vi "test_struct_ads_volume.vi"() -> ()   [LabVIEW 2017]
doc: "Minimal example that demonstrates functions implemented in the SorpPropLib for adsorption working pairs based on the volumetric approach and using the vapor pressure as additional property."
panel:
  out "Der. of loading wrt. pressure":cluster{dbl[], dbl[]}[](graph)
  out "Der. of loading wrt. temperature":cluster{dbl[], dbl[]}[](graph)
  out "Der. of pressure wrt. loading":cluster{dbl[], dbl[]}[](graph)
  out "Der. of pressure wrt. temperature":cluster{dbl[], dbl[]}[](graph)
  out "Temperature":cluster{dbl[], dbl[]}[](graph)
  out "Pressure":cluster{dbl[], dbl[]}[](graph)
  out "Loading":cluster{dbl[], dbl[]}[](graph)
  in  "WorkingPair (Input)":T1={"no_iso"=1, "no_p_sat"=1, "path_db"="D:\\Driesel\\SorpLibLocal\\labview_wrapper\\data\\json\\sorpproplib.json", "wp_as"="silica gel pellet", "wp_st"="123", "wp_iso"="DubininArctan1", "wp_rf"="Water", "rf_rhol"="SaturatedLiquidDensity_EoS1", "no_rhol"=1, "rf_psat"="VaporPressure_EoS1"}
  in  "Temperature in K (Input)":dbl=300.0
  in  "Pressure in Pa (Input)":dbl=1000.0
  # "Increase pressure by 5000 Pa in steps of 1 Pa."
  # "Path to database"
  # "Name of sorbent"
  # "Name of sub-type of sorbent"
  # "Name of refrigerant"
  # "Name of isotherm"
  # "ID of isotherm"
  # "Name of calculation approach for vapor pressure"
  # "ID of vapor pressure equation"
  # "Name of calculation approach for liquid density"
  # "ID of liquid density equation"
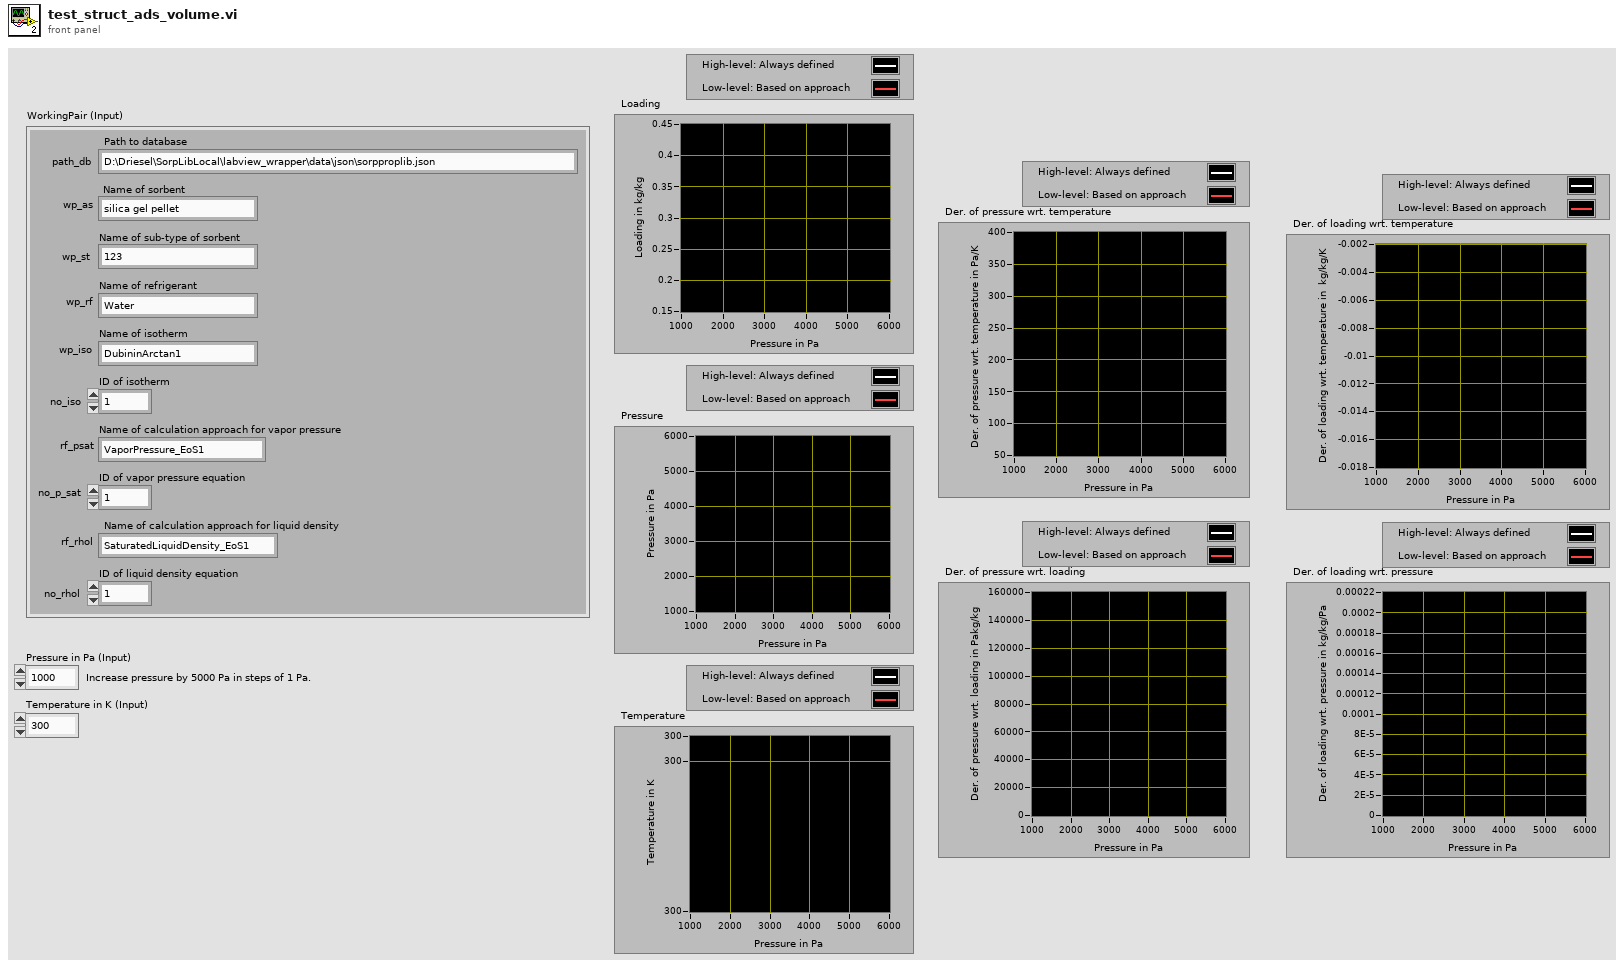
[diagram p1: front panel]
types:
  T1 = cluster{"no_iso":i32, "no_p_sat":i32, "path_db":string, "wp_as":string, "wp_st":string, "wp_iso":string, "wp_rf":string, "rf_rhol":string, "no_rhol":i32, "rf_psat":string}
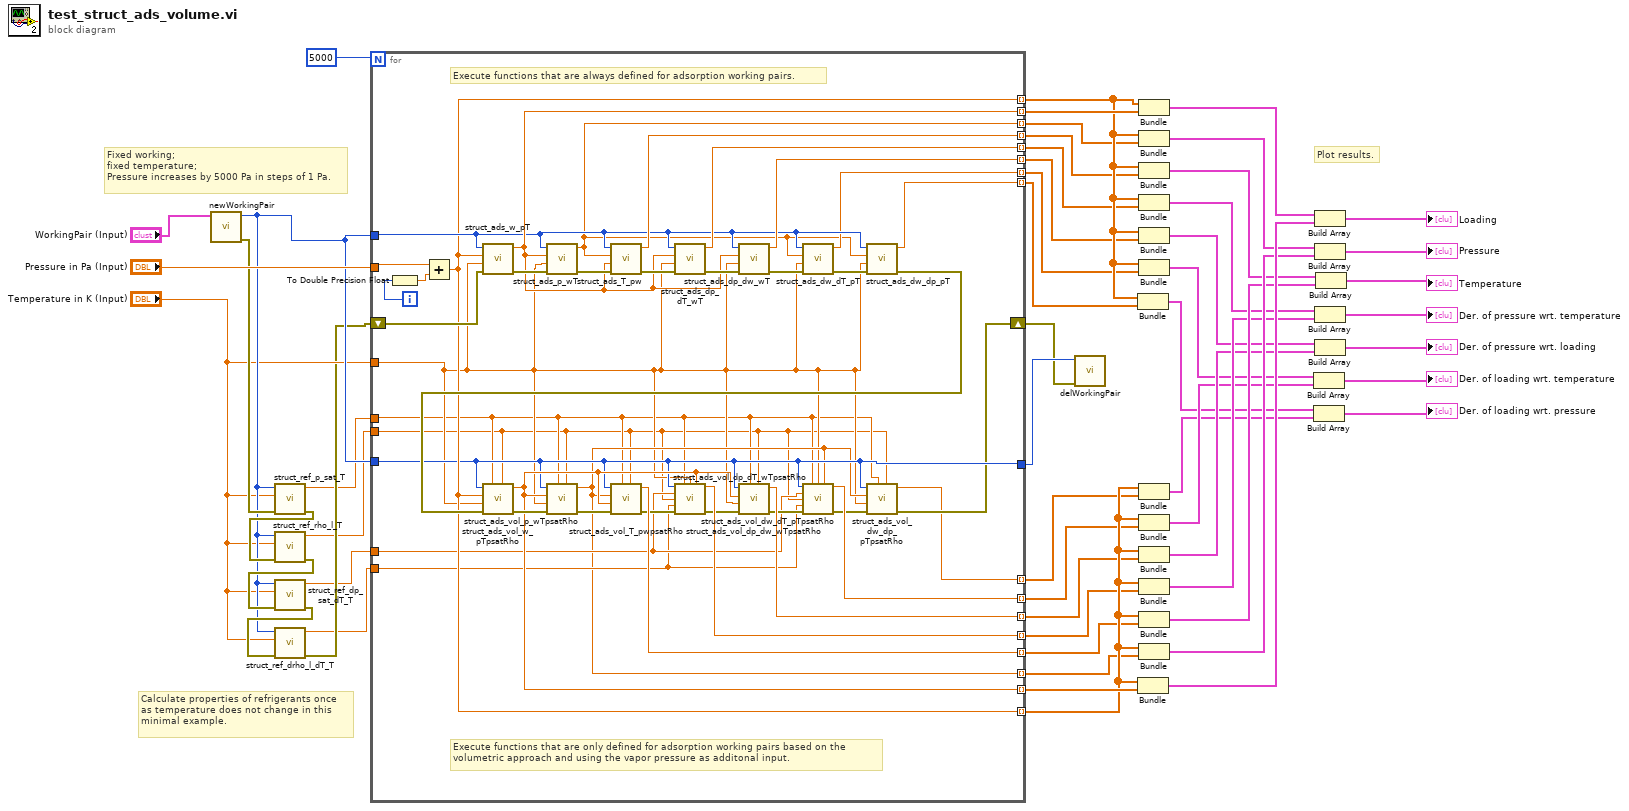
[diagram p0: block diagram]
diagram:
  # "Calculate properties of refrigerants once\nas temperature does not change in this\nminimal example."
  # "Plot results."
  # "Fixed working;\nfixed temperature;\nPressure increases by 5000 Pa in steps of 1 Pa."
  n1 = call "newWorkingPair.vi"("WorkingPair (Input)"="WorkingPair (Input)") -> ("Error (Output)"=w11:errorcluster, "workingPair"=w7:i64)  [unwired: 9 in]
  n2 = call "struct_ref_p_sat_T.vi"("Error (Input)"=w11, "Temperature in K (Input)"="Temperature in K (Input)", "Reference working pair (Input)"=w7) -> ("Error (Output)"=w10:errorcluster, "Saturation pressure in Pa (Output)"=w4:dbl)  [unwired: 7 in]
  n3 = call "struct_ref_rho_l_T.vi"("Error (Input)"=w10, "Temperature in K (Input)"="Temperature in K (Input)", "Reference working pair (Input)"=w7) -> ("Error (Output)"=w9:errorcluster, "Saturated liquid density in kg/m3 (Output)"=w3:dbl)  [unwired: 7 in]
  n4 = call "struct_ref_dp_sat_dT_T.vi"("Error (Input)"=w9, "Temperature in K (Input)"="Temperature in K (Input)", "Reference working pair (Input)"=w7) -> ("Error (Output)"=w8:errorcluster, "Der. of saturation pressure wrt temperature in Pa/K (Output)"=w2:dbl)  [unwired: 7 in]
  n5 = call "struct_ref_drho_l_dT_T.vi"("Error (Input)"=w8, "Temperature in K (Input)"="Temperature in K (Input)", "Reference working pair (Input)"=w7) -> ("Error (Output)"=w5:errorcluster, "Der. of saturated liquid density wrt temperature in kg/m3/K (Output)"=w1:dbl)  [unwired: 7 in]
  n6 = for {
    N: 5000 -> [_]
    tunnel: "Pressure in Pa (Input)" -> [w93]
    tunnel: "Temperature in K (Input)" -> [w59]
    tunnel: w7 -> [w79]
    shift-right: [w55] -> w12
    shift-left: w5 -> [w90]
    tunnel: [w88] -> w48 mode=indexing
    tunnel: [w74] -> w50 mode=indexing
    tunnel: [w81] -> w51 mode=indexing
    tunnel: [w76] -> w49 mode=indexing
    tunnel: [w86] -> w47 mode=indexing
    tunnel: [w83] -> w46 mode=indexing
    tunnel: [w78] -> w44 mode=indexing
    tunnel: [w77] -> w45 mode=indexing
    tunnel: w7 -> [w61]
    tunnel: [w67] -> w43 mode=indexing
    tunnel: [w74] -> w42 mode=indexing
    tunnel: [w60] -> w41 mode=indexing
    tunnel: [w72] -> w40 mode=indexing
    tunnel: [w70] -> w29 mode=indexing
    tunnel: [w66] -> w26 mode=indexing
    tunnel: [w62] -> w22 mode=indexing
    tunnel: [w54] -> w21 mode=indexing
    tunnel: [w61] -> w13
    tunnel: w4 -> [w58]
    tunnel: w3 -> [w57]
    tunnel: w2 -> [w64]
    tunnel: w1 -> [w63]
    i -> [w92]
    # "Execute functions that are only defined for adsorption working pairs based on the\nvolumetric approach and using the vapor pressure as additonal input."
    # "Execute functions that are always defined for adsorption working pairs."
    n7 = To Double Precision Float(number=w92) -> (double precision float=w91:dbl)
    n8 = Add(x=w93, y=w91) -> (x+y=w74:dbl)
    n9 = call "struct_ads_w_pT.vi"("Error (Input)"=w90, "Temperature in K (Input)"=w59, "Pressure in Pa (Input)"=w74, "Reference working pair (Input)"=w79) -> ("Error (Output)"=w89:errorcluster, "Loading in kg/kg (Output)"=w81:dbl)  [unwired: 6 in]
    n10 = call "struct_ads_p_wT.vi"("Error (Input)"=w89, "Temperature in K (Input)"=w59, "Loading in kg/kg (Input)"=w81, "Reference working pair (Input)"=w79) -> ("Error (Output)"=w87:errorcluster, "Pressure in Pa (Output)"=w76:dbl)  [unwired: 6 in]
    n11 = call "struct_ads_T_pw.vi"("Error (Input)"=w87, "Loading in kg/kg (Input)"=w81, "Pressure in Pa (Input)"=w76, "Reference working pair (Input)"=w79) -> ("Error (Output)"=w85:errorcluster, "Temperature in K (Output)"=w88:dbl)  [unwired: 6 in]
    n12 = call "struct_ads_dp_dT_wT.vi"("Error (Input)"=w85, "Temperature in K (Input)"=w59, "Loading in kg/kg (Input)"=w81, "Reference working pair (Input)"=w79) -> ("Error (Output)"=w84:errorcluster, "Der. of pressure wrt. temperature in Pa/K (Output)"=w86:dbl)  [unwired: 6 in]
    n13 = call "struct_ads_dp_dw_wT.vi"("Error (Input)"=w84, "Temperature in K (Input)"=w59, "Loading in kg/kg (Input)"=w81, "Reference working pair (Input)"=w79) -> ("Error (Output)"=w82:errorcluster, "Der. of pressure wrt. loading in Pakg/kg (Output)"=w83:dbl)  [unwired: 6 in]
    n14 = call "struct_ads_dw_dT_pT.vi"("Error (Input)"=w82, "Temperature in K (Input)"=w59, "Pressure in Pa (Input)"=w76, "Reference working pair (Input)"=w79) -> ("Error (Output)"=w80:errorcluster, "Der. of loading wrt. temperature in kg/kg/K (Output)"=w78:dbl)  [unwired: 6 in]
    n15 = call "struct_ads_dw_dp_pT.vi"("Error (Input)"=w80, "Temperature in K (Input)"=w59, "Pressure in Pa (Input)"=w76, "Reference working pair (Input)"=w79) -> ("Error (Output)"=w75:errorcluster, "Der. of loading wrt. pressure in kg/kg/Pa (Output)"=w77:dbl)  [unwired: 6 in]
    n16 = call "struct_ads_vol_w_pTpsatRho.vi"("Saturated liquid density of adsorpt in kg/m3 (Input)"=w57, "Saturation pressure in Pa (Input)"=w58, "Error (Input)"=w75, "Temperature in K (Input)"=w59, "Pressure in Pa (Input)"=w74, "Reference working pair (Input)"=w61) -> ("Error (Output)"=w73:errorcluster, "Loading in kg/kg (Output)"=w67:dbl)  [unwired: 4 in]
    n17 = call "struct_ads_vol_p_wTpsatRho.vi"("Density of adsorpt in kg/m3 (Input)"=w57, "Saturation pressure in Pa (Input)"=w58, "Error (Input)"=w73, "Temperature in K (Input)"=w59, "Loading in kg/kg (Input)"=w67, "Reference working pair (Input)"=w61) -> ("Error (Output)"=w71:errorcluster, "Pressure in Pa (Output)"=w60:dbl)  [unwired: 4 in]
    n18 = call "struct_ads_vol_T_pwpsatRho.vi"("Density of adsorpt in kg/m3 (Input)"=w57, "Saturation pressure in Pa (Input)"=w58, "Error (Input)"=w71, "Loading in kg/kg (Input)"=w67, "Pressure in Pa (Input)"=w60, "Reference working pair (Input)"=w61) -> ("Error (Output)"=w69:errorcluster, "Equilibrium temperature in K (Output)"=w72:dbl)  [unwired: 4 in]
    n19 = call "struct_ads_vol_dp_dT_wTpsatRho.vi"("Reference working pair (Input)"=w61, "Saturation pressure in Pa (Input)"=w58, "Temperature in K (Input)"=w59, "Loading in kg/kg (Input)"=w67, "Der. of saturation pressure wrt. temperature in Pa/K (Input)"=w64, "Density of adsorpt in kg/m3 (Input)"=w57, "Der. of density of adsorpt wrt. temperature in kg/m3/K (Input)"=w63, "Error (Input)"=w69) -> ("Der. of equilibrium pressure wrt. temperature in Pa/K (Output)"=w70:dbl, "Error (Output)"=w68:errorcluster)  [unwired: 6 in]
    n20 = call "struct_ads_vol_dp_dw_wTpsatRho.vi"("Density of adsorpt in kg/m3 (Input)"=w57, "Saturation pressure in Pa (Input)"=w58, "Error (Input)"=w68, "Temperature in K (Input)"=w59, "Loading in kg/kg (Input)"=w67, "Reference working pair (Input)"=w61) -> ("Error (Output)"=w65:errorcluster, "Der. of equilibrium pressure wrt. loading in Pakg/kg (Output)"=w66:dbl)  [unwired: 4 in]
    n21 = call "struct_ads_vol_dw_dT_pTpsatRho.vi"("Reference working pair (Input)"=w61, "Saturation pressure in Pa (Input)"=w58, "Temperature in K (Input)"=w59, "Pressure Pa (Input)"=w60, "Der. of saturation pressure wrt. temperature in Pa/K (Input)"=w64, "Density of adsorpt in kg/m3 (Input)"=w57, "Der. of density of adsorpt wrt. temperature in kg/m3/K (Input)"=w63, "Error (Input)"=w65) -> ("Der. of loading wrt. temperature in kg/kg/K (Output)"=w62:dbl, "Error (Output)"=w56:errorcluster)  [unwired: 6 in]
    n22 = call "struct_ads_vol_dw_dp_pTpsatRho.vi"("Density of adsorpt in kg/m3 (Input)"=w57, "Saturation pressure in Pa (Input)"=w58, "Error (Input)"=w56, "Temperature in K (Input)"=w59, "Pressure in Pa (Input)"=w60, "Reference working pair (Input)"=w61) -> ("Error (Output)"=w55:errorcluster, "Der. of loading wrt. pressure in kg/kg/Pa (Output)"=w54:dbl)  [unwired: 4 in]
  }
  n23 = call "delWorkingPair.vi"("Error (Input)"=w12, "workingPair"=w13) -> ()  [unwired: 9 in, 1 out]
  n24 = Bundle(w50, w45) -> (w18:cluster{dbl[], dbl[]})  [unwired: 1 in]
  n25 = Bundle(w42, w43) -> (w38:cluster{dbl[], dbl[]})  [unwired: 1 in]
  n26 = Bundle(w50, w51) -> (w39:cluster{dbl[], dbl[]})  [unwired: 1 in]
  n27 = Bundle(w50, w49) -> (w37:cluster{dbl[], dbl[]})  [unwired: 1 in]
  n28 = Bundle(w50, w48) -> (w35:cluster{dbl[], dbl[]})  [unwired: 1 in]
  n29 = Bundle(w50, w47) -> (w33:cluster{dbl[], dbl[]})  [unwired: 1 in]
  n30 = Bundle(w50, w46) -> (w25:cluster{dbl[], dbl[]})  [unwired: 1 in]
  n31 = Bundle(w50, w44) -> (w20:cluster{dbl[], dbl[]})  [unwired: 1 in]
  n32 = Bundle(w42, w21) -> (w17:cluster{dbl[], dbl[]})  [unwired: 1 in]
  n33 = Bundle(w42, w22) -> (w19:cluster{dbl[], dbl[]})  [unwired: 1 in]
  n34 = Bundle(w42, w26) -> (w24:cluster{dbl[], dbl[]})  [unwired: 1 in]
  n35 = Bundle(w42, w29) -> (w28:cluster{dbl[], dbl[]})  [unwired: 1 in]
  n36 = Bundle(w42, w40) -> (w34:cluster{dbl[], dbl[]})  [unwired: 1 in]
  n37 = Bundle(w42, w41) -> (w36:cluster{dbl[], dbl[]})  [unwired: 1 in]
  n38 = Build Array(w20, w19) -> (→"Der. of loading wrt. temperature":cluster{dbl[], dbl[]}[])
  n39 = Build Array(w18, w17) -> (→"Der. of loading wrt. pressure":cluster{dbl[], dbl[]}[])
  n40 = Build Array(w39, w38) -> (→"Loading":cluster{dbl[], dbl[]}[])
  n41 = Build Array(w37, w36) -> (→"Pressure":cluster{dbl[], dbl[]}[])
  n42 = Build Array(w33, w28) -> (→"Der. of pressure wrt. temperature":cluster{dbl[], dbl[]}[])
  n43 = Build Array(w25, w24) -> (→"Der. of pressure wrt. loading":cluster{dbl[], dbl[]}[])
  n44 = Build Array(w35, w34) -> (→"Temperature":cluster{dbl[], dbl[]}[])
